vi "update.vi"(0 "Display State In":T1, 9 "Container State":T2, 11 "error in (no error)":errorcluster) -> (4 "Display State Out":T1, 15 "error out":errorcluster)   [LabVIEW 2010, in "XSettings.xctl"]
uses:
  XSettings.xctl
  <vilib>/_xctls/Container State.ctl
  state.ctl
  classes/GenericComponent/GenericComponent/GenericComponent.lvclass
  data.ctl
  <vilib>/_xctls/XControlSupport.lvlib
panel:
  # "Add Controls & Indicators that form the parameters of the method here. Hook them to the connector pane. Do not delete the controls & indicators that are already hooked to the connector pane.\n \nTo setup the parameters  for this method, right click on this item in the Project Tree & select \"Configure Method...\"."
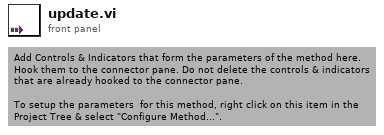
[diagram p1: front panel]
types:
  T1 = typedef "XSettings.xctl/state.ctl" = cluster{"error":errorcluster, "user-defined?":bool, "control refs":cluster{"settings combo":refnum<vi>}}
  T2 = typedef "XControlSupport.lvlib/Container State.ctl" = cluster{"Indicator?":bool, "Run Mode?":bool, " Refnum":refnum<vi>}
  T3 = typedef "XSettings.xctl/data.ctl" = refnum<class "GenericComponent.lvclass">
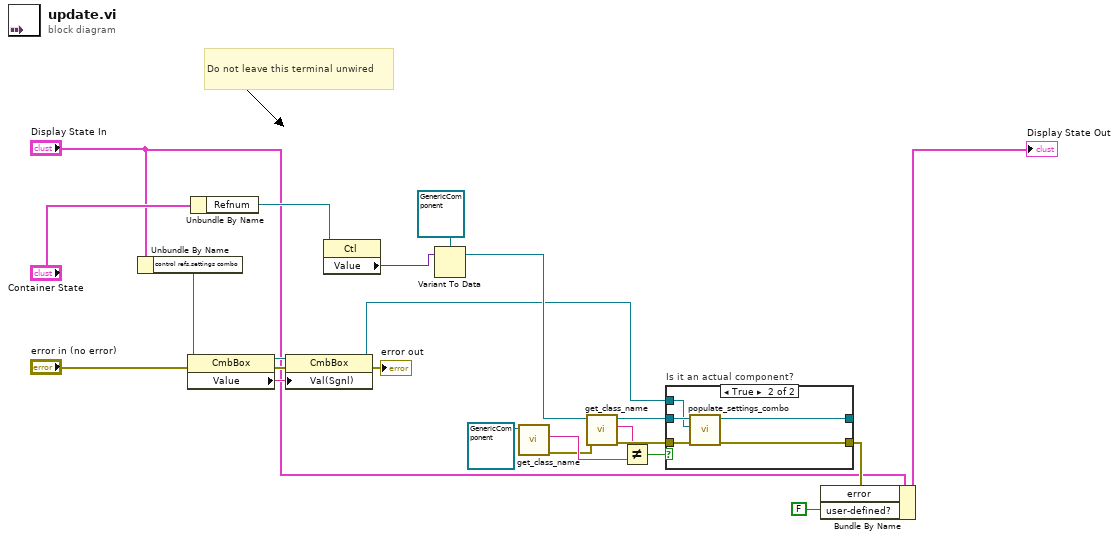
[diagram p0: block diagram]
diagram:
  # "Do not leave this terminal unwired"
  n1 = Unbundle By Name("Display State In") -> ("control refs.settings combo"=w23:refnum<vi>)
  n2 = property class="CmbBox"(reference=w23, error in="error in (no error)") -> (reference out=w22:refnum<vi>, error out=w21:errorcluster, "Value"=w20:string)
  n3 = Unbundle By Name("Container State") -> ("Refnum"=w7:refnum<vi>)
  n4 = property class="CmbBox"(reference=w22, error in=w21, "Val(Sgnl)"=w20) -> (reference out=w1:refnum<vi>, error out=→"error out":errorcluster)
  n5 = property class="Ctl"(reference=w7) -> ("Value"=w6:variant)  [unwired: 1 in, 2 out]
  n6 = Variant To Data(Variant=w6, type=T3 refnum ("component")) -> (data=w4:T3)  [unwired: 1 in, 1 out]
  n7 = call-dynamic "get_class_name.vi"("GenericPlugin in"=refnum<class "GenericComponent.lvclass"> refnum ("GenericComponent.lvclass")) -> ("error out"=w11:errorcluster, "class name"=w12:string)  [unwired: 6 in, 3 out]
  n8 = call-dynamic "get_class_name.vi"("error in (no error)"=w11, "GenericPlugin in"=w4) -> ("error out"=w14:errorcluster, "class name"=w13:string, "GenericPlugin out"=w16:T3)  [unwired: 5 in, 2 out]
  n9 = Not Equal?(x=w13, y=w12) -> (x != y?=w15:bool)
  n10 = case "Is it an actual component?" shown="True" w15 {
    tunnel: [w25 w30] -> _
    tunnel: w16 -> [w25 w29]
    tunnel: w14 -> [w24 w27]
    tunnel: [w24 w28] -> w10
    tunnel: w1 -> [_ w26]
    frame False {
      # "It's just a GenericComponent..."
    }
    frame True {
      n11 = call-dynamic "populate_settings_combo.vi"("error in (no error)"=w27, "combo box ref"=w26, "GenericPlugin in"=w29) -> ("error out"=w28:errorcluster, "GenericPlugin out"=w30:T3)  [unwired: 7 in]
    }
  }
  n12 = Bundle By Name(cluster="Display State In", "error"=w10, "user-defined?"=FALSE) -> (→"Display State Out":T1)
